vi "FTW-DevUtil-RegisterProbes.vi"() -> ()   [LabVIEW 2015]
panel:
  out "error out":errorcluster
  out "Probes Added":string[](array[string])
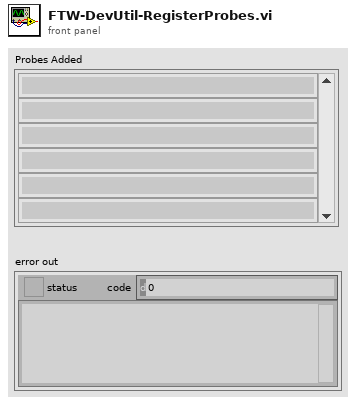
[diagram p1: front panel]
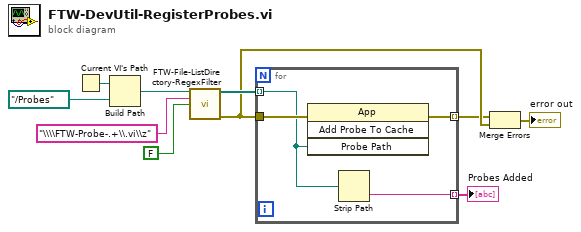
[diagram p0: block diagram]
diagram:
  n1 = Current VI's Path() -> (path=w9:path)
  n2 = Build Path(base path=w9, name or relative path=path "../Probes") -> (appended path=w7:path)
  n3 = call "FTW-File-ListDirectory-RegexFilter.vi"("Directory to Search"=w7, "Filename Regex Filter"="\\\\FTW-Probe-.+\\.vi\\z", "Treat LLBs as Folders?"=FALSE) -> ("Matching Filepaths"=w6:path[], "error out"=w5:errorcluster)  [unwired: 9 in, 2 out]
  n4 = for {
    tunnel: w5 -> [w14]
    tunnel: w6 -> [w12] mode=indexing
    tunnel: [w13] -> w4 mode=indexing
    tunnel: [w11] -> w2 mode=indexing
    n5 = invoke class="App" method="Add Probe To Cache"(error in=w14, "Probe Path"=w12) -> (error out=w13:errorcluster)  [unwired: 2 in, 3 out]
    n6 = Strip Path(path=w12) -> (name=w11:string)  [unwired: 1 out]
  }
  "Probes Added" <- w2
  n7 = Merge Errors(w4, w5) -> (→"error out":errorcluster)
